vi "1D STR Array_DeleteCellsWithSpecifiedValue_ArrayInput.vi"(1 "CellValueToBeDeleted":string[](array[string]), 2 "1D STR Array.IN":string[](array[string])=["", ""]) -> (6 "1D STR Array.OUT":string[](array[string]))   [LabVIEW 2020]
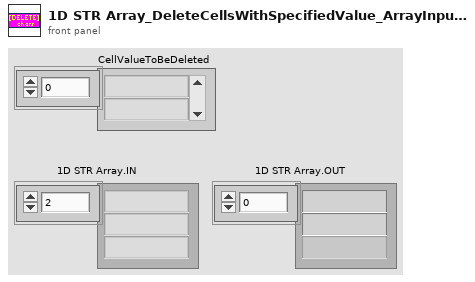
[diagram p1: front panel]
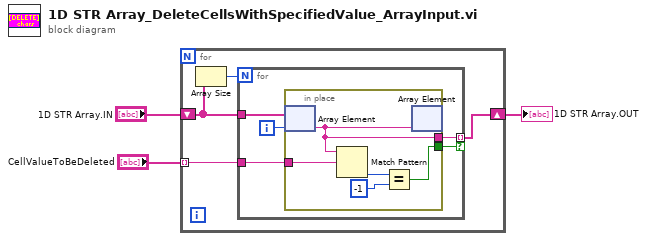
[diagram p0: block diagram]
diagram:
  n1 = for {
    tunnel: "CellValueToBeDeleted" -> [w4] mode=indexing
    shift-right: [w5] -> w2
    shift-left: "1D STR Array.IN" -> [w6]
    n2 = Array Size(array=w6) -> (size(s)=w7:i32)
    n3 = for {
      N: w7 -> [_]
      tunnel: w6 -> [w12]
      tunnel: [w10] -> w5 mode=indexing if=w8
      tunnel: w4 -> [w9]
      i -> [w11]
      n4 = in-place {
        in-place-border: [w16] -> w10
        in-place-border: w9 -> [w15]
        in-place-border: [w17] -> w8
        n5 = in-place-array #1(w12, w11) -> (w16:string)
        n6 = Match Pattern(string=w16, regular expression=w15) -> (offset past match=w14:i32)  [unwired: 1 in, 3 out]
        n7 = Equal?(x=w14, y=-1) -> (x = y?=w17:bool)
        n8 = in-place-array #1(w16) -> ()  [unwired: 2 out]
      }
    }
  }
  "1D STR Array.OUT" <- w2
